vi "Configure Signal Polarity.vi"(7 "Enable Output Connector (T: Enable)":bool=TRUE, 8 "error in (no error)":errorcluster, 9 "Polarity (0: Positive)":i32(ring) items=["Positive", "Negative"], 10 "Connector (0: Burst Gate In connector)":i32(ring) items=["Burst Gate In", "Data Clock", "Data", "Symbol Sync", "Data Clock  Out", "Data Out", "Symbol Sync Out"], 11 "VISA resource name":refnum<visa-resource-name>) -> (0 "error out":errorcluster, 3 "VISA resource name out":refnum<visa-resource-name>)   [LabVIEW 2014, in "Agilent PSG MXG Series.lvlib"]
doc: "Configures the polarity of the TTL input signal at the specified connector.\n\n<B>Notes:</B>\n(1) This VI is valid only in N5172B, N5182B.\n\n(2) For N5172B, this VI is valid only when the instrument installs <B>Option 653</B> or <B>Option 655</B>.\n\n(3) For N5182B, this VI is valid only when the instrument installs <B>Option 656</B> or <B>Option 657</B>."
uses:
  Agilent PSG MXG Series.lvlib
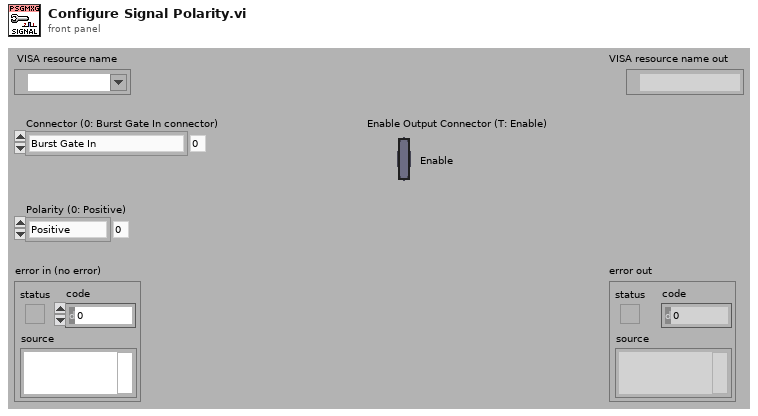
[diagram p1: front panel]
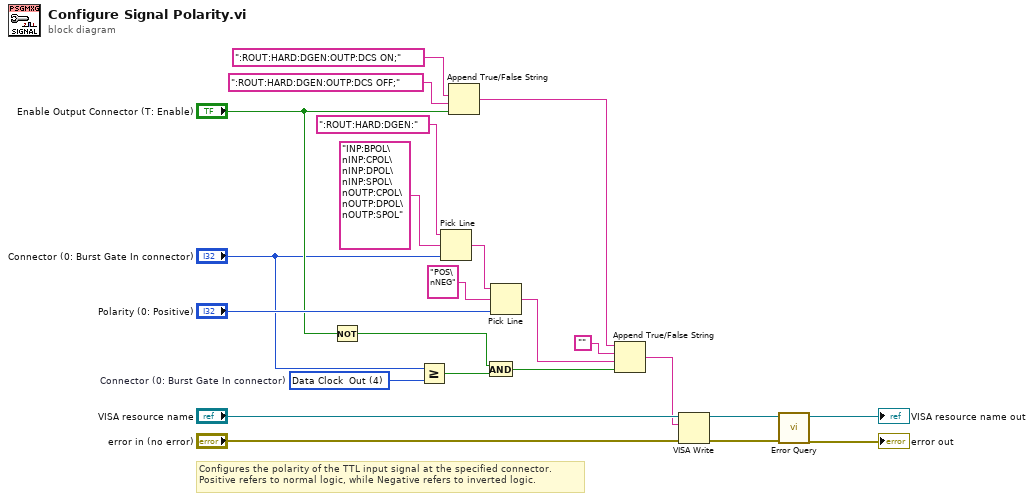
[diagram p0: block diagram]
diagram:
  w8 = 4 items=["Burst Gate In", "Data Clock", "Data", "Symbol Sync", "Data Clock  Out", "Data Out", "Symbol Sync Out"]  # Connector (0: Burst Gate In connector)
  # "Configures the polarity of the TTL input signal at the specified connector.\nPositive refers to normal logic, while Negative refers to inverted logic."
  n1 = Not(x="Enable Output Connector (T: Enable)") -> (.not. x?=w11:bool)
  n2 = Greater Or Equal?(x="Connector (0: Burst Gate In connector)", y=w8) -> (x >= y?=w7:bool)
  n3 = Pick Line(string ("")=":ROUT:HARD:DGEN:", multi-line string="INP:BPOL\nINP:CPOL\nINP:DPOL\nINP:SPOL\nOUTP:CPOL\nOUTP:DPOL\nOUTP:SPOL", line index="Connector (0: Burst Gate In connector)") -> (output string=w2:string)
  n4 = Append True/False String(1:"Enable Output Connector (T: Enable)", 2:":ROUT:HARD:DGEN:OUTP:DCS OFF;", 3:":ROUT:HARD:DGEN:OUTP:DCS ON;") -> (0:w6:string)  [unwired: 1 out]
  n5 = And(x=w11, y=w7) -> (x .and. y?=w12:bool)
  n6 = Pick Line(string ("")=w2, multi-line string="POS\nNEG", line index="Polarity (0: Positive)") -> (output string=w1:string)
  n7 = Append True/False String(1:w12, 2:w1, 3:"", 4:w6) -> (0:w5:string)
  n8 = VISA Write(VISA resource name="VISA resource name", write buffer=w5, error in (no error)="error in (no error)") -> (VISA resource name out=w21:refnum<visa-resource-name>, error out=w20:errorcluster)  [unwired: 1 out]
  n9 = call "Error Query.vi"("error in (no error)"=w20, "VISA resource name"=w21) -> ("error out"=→"error out":errorcluster, "VISA resource name out"=→"VISA resource name out":refnum<visa-resource-name>)  [unwired: 8 out]
